vi "Actor Core.vi"(8 "error in":errorcluster, 11 "Server in":refnum<class "Server.lvclass">) -> (0 "error out":errorcluster, 3 "Actor out":refnum<class "Actor.lvclass">)   [LabVIEW 2018, in "Server.lvlib" / "Server.lvclass"]
doc: "(<B>Filename</B>: Actor Framework.lvlib:Actor.lvclass:Actor Core.vi)\n\nReceives messages to the actor, reacts to them, and initiates any error handling that may shut the actor down.\n\nDescendant classes may override this VI to append parallel tasks for the actor to complete while it handles messages. Overrides use the Call Parent Method node."
uses:
  Server.lvclass
  C:/Program Files (x86)/National Instruments/LabVIEW 2018/vi.lib/ActorFramework/Actor/Actor.lvclass
  <vilib>/ActorFramework/Actor/Actor.lvclass
  <vilib>/ActorFramework/Actor/Actor.lvclass/Actor.ctl
  <vilib>/ActorFramework/Message Enqueuer/Message Enqueuer.lvclass/Message Enqueuer.ctl
  Server.lvclass/Server.ctl
  Server Messages/Send Global Chat Msg/Send Global Chat Msg.lvclass/Send Global Chat Msg.ctl
  <vilib>/ActorFramework/Message Enqueuer/Init from Existing Queue.vi
  <vilib>/ActorFramework/Message Enqueuer/Enqueue.vi
  Server Messages/Launch New Chat Window Msg/Launch New Chat Window Msg.lvclass
  C:/Program Files (x86)/National Instruments/LabVIEW 2018/vi.lib/ActorFramework/Message/Message.lvclass
  Server Messages/Send Global Chat Msg/Send Global Chat Msg.lvclass
  <vilib>/ActorFramework/Stop Msg/Stop Msg.lvclass
  <vilib>/ActorFramework/Message Priority Queue/Priority Enqueue.vi
  <vilib>/ActorFramework/Message Enqueuer/Message Enqueuer.lvclass
panel:
  in  "Message":string
  in  "Send Global Chat":bool
  in  "Launch Chat Window":bool
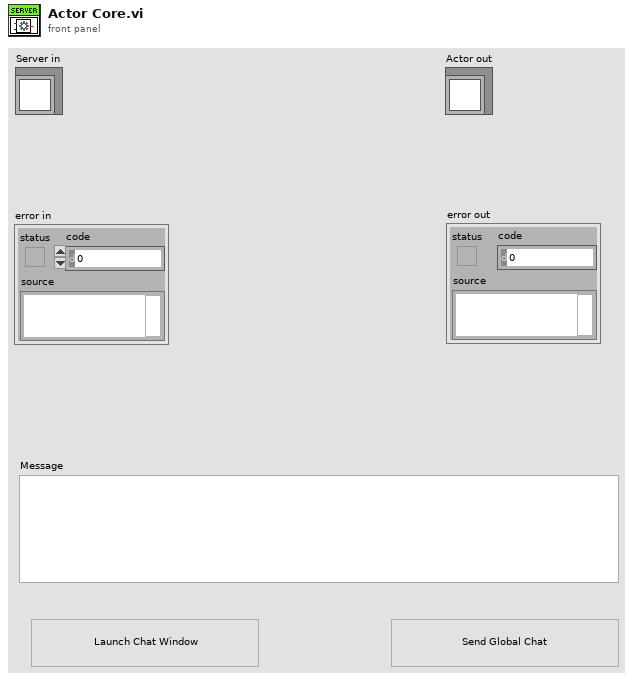
[diagram p1: front panel]
types:
  T1 = enum32{"Invalid", "Standard", "Closed", "Hidden", "Minimized", "Maximized"}
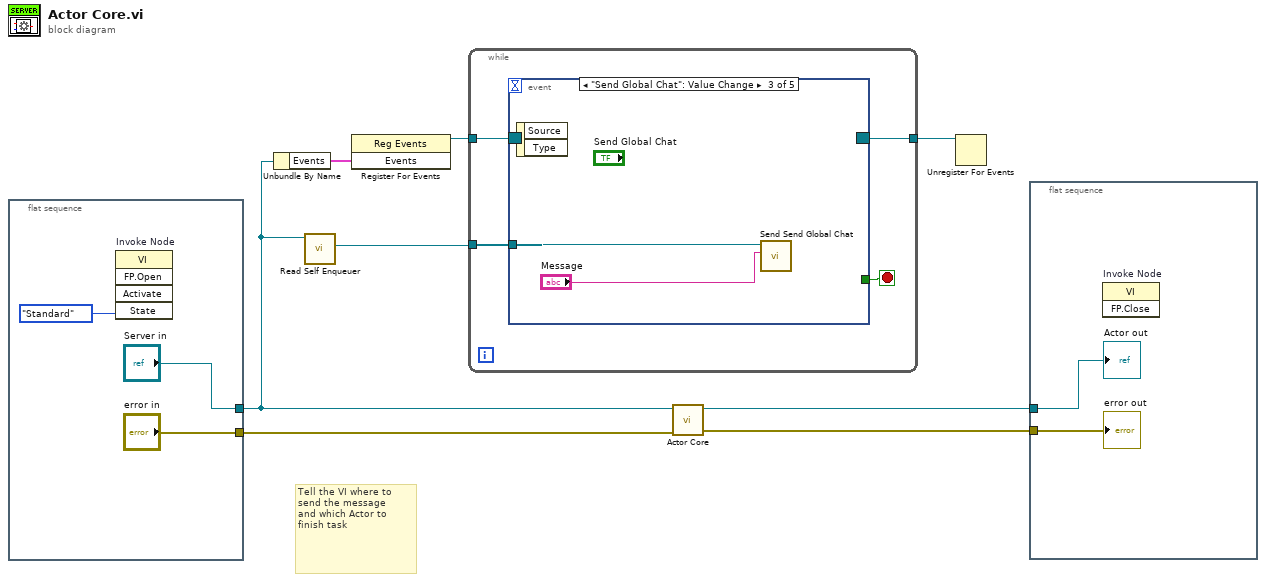
[diagram p0: block diagram]
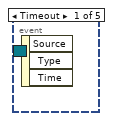
[diagram p2: hidden frame]
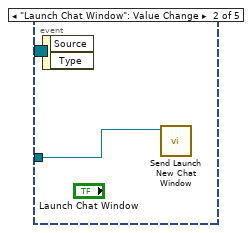
[diagram p3: hidden frame]
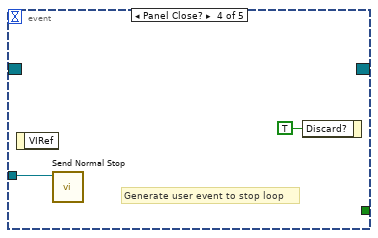
[diagram p4: hidden frame]
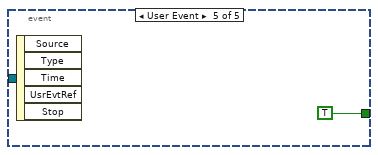
[diagram p5: hidden frame]
diagram:
  # "Tell the VI where to send the message\nand which Actor to finish task"
  n1 = flat-sequence {
    tunnel: ["error in"] -> w6
    tunnel: ["Server in"] -> w4
    frame #0 {
      n2 = invoke on="Invoke Node" class="VI" method="FP.Open"("State"=T1."Standard") -> ()  [unwired: 4 in, 5 out]
    }
  }
  n3 = Unbundle By Name(w4) -> ("Events"=w3:cluster{"Stop":refnum<user-event>})
  n4 = call <vilib>:"Read Self Enqueuer.vi"("Actor"=w4) -> ("Self Enqueuer"=w5:refnum<class "Message Enqueuer.lvclass">)  [unwired: 10 in]
  n5 = register-events(w3) -> (reference out=w2:refnum<event-registration>)  [unwired: 2 in, 1 out]
  n6 = while {
    tunnel: w5 -> [w15]
    tunnel: w2 -> [w14]
    tunnel: [w12] -> w1
    stop <- w13 stop-if-true
    n7 = event shown="[2] \"Send Global Chat\": Value Change" {
      selector: w14 -> [_ _ _ _ _]
      dyn-events: [_ _ _ _ _] -> w12
      timeout: _ -> [_ _ _ _ _]
      tunnel: w15 -> [_ w16 w18 w19 _]
      tunnel: [_ _ _ _ TRUE] -> w13
      event Timeout {
        n8 = event-data() -> ()  [unwired: 1 in, 3 out]
      }
      event "Launch Chat Window": Value Change {
        n9 = event-data() -> ()  [unwired: 1 in, 2 out]
        n10 = call "Send Launch New Chat Window.vi"("Message Enqueuer"=w16) -> ()  [unwired: 9 in, 2 out]
      }
      event "Send Global Chat": Value Change {
        n11 = event-data() -> ()  [unwired: 1 in, 2 out]
        n12 = call "Send Send Global Chat.vi"("Message"="Message", "Message Enqueuer"=w18) -> ()  [unwired: 8 in, 2 out]
      }
      event Panel Close? {
        # "Generate user event to stop loop"
        n13 = event-data() -> ()  [unwired: 1 in, 1 out]
        n14 = call <vilib>:"Send Normal Stop.vi"("Message Enqueuer"=w19) -> ()  [unwired: 10 in, 1 out]
        n15 = event-data("Discard?"=TRUE) -> ()  [unwired: 1 in, 1 out]
      }
      event User Event {
        n16 = event-data() -> ()  [unwired: 1 in, 5 out]
      }
    }
  }
  n17 = call-parent "Actor Core.vi"("error in"=w6, "Actor in"=w4) -> ("error out"=w8:errorcluster, "Actor out"=w7:refnum<class "Actor.lvclass">)  [unwired: 8 in]
  n18 = Unregister For Events(event registration refnum=w1) -> ()  [unwired: 1 in, 1 out]
  n19 = flat-sequence {
    tunnel: w8 -> [w23]
    tunnel: w7 -> [w22]
    frame #0 {
      n20 = invoke on="Invoke Node" class="VI" method="FP.Close"() -> ()  [unwired: 3 in, 3 out]
      "error out" <- w23
      "Actor out" <- w22
    }
  }
